vi "clear_buffers.vi"(8 "error in (no error)":errorcluster, 11 "FPGAWrapperAN110607Galvo in":refnum<class "FPGAWrapperAN110607Galvo.lvclass">) -> (0 "error out":errorcluster, 3 "FPGAWrapperAN110607Galvo out":refnum<class "FPGAWrapperAN110607Galvo.lvclass">)   [LabVIEW 2010, in "FPGAWrapperAN110607Galvo.lvclass"]
uses:
  FPGAWrapperAN110607Galvo.lvclass
  <vilib>/rvi/interface/nirviMethod/nirviMethod.xnode
  FPGA_VI_ref.ctl
  <vilib>/rvi/interface/common/niFpgaNodeNameForErrorReporting.ctl
  <vilib>/rvi/errors/niLvFpgaWhatHappensToTopLevelVI.ctl
  <vilib>/Utility/error.llb/Error Cluster From Error Code.vi
  <vilib>/rvi/errors/niLvFpgaAdjustHostInterfaceError.vi
  NiFpgaLv.dll
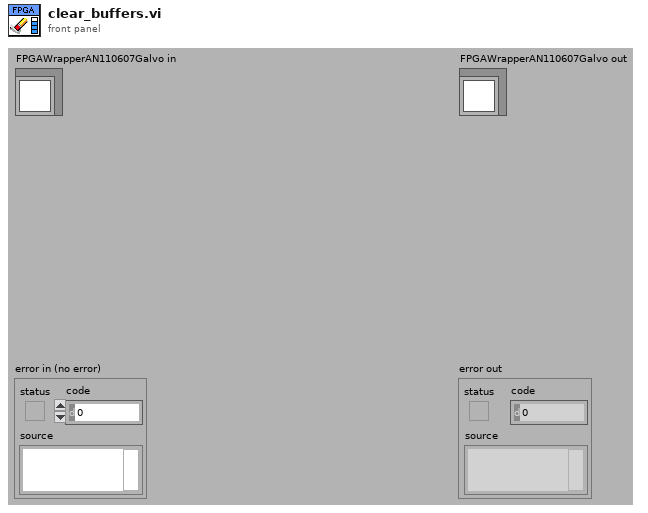
[diagram p1: front panel]
types:
  T1 = typedef "niFpgaNodeNameForErrorReporting.ctl" = enum16{"Open FPGA VI Reference", "Read/Write Control", "Invoke Method: Abort", "Invoke Method: Acknowledge IRQ", "Invoke Method: Download", "Invoke Method: FIFO.Configure", "Invoke Method: FIFO.Read", "Invoke Method: FIFO.Start", "Invoke Method: FIFO.Stop", "Invoke Method: FIFO.Write", "Invoke Method: Reset", "Invoke Method: Run", "Invoke Method: Wait on IRQ", "Close FPGA VI Reference"}
  T2 = typedef "niLvFpgaWhatHappensToTopLevelVI.ctl" = enum16{"top level VI scripted behind XNode", "top level VI inlined behind XNode"}
  T3 = typedef "FPGAWrapperAN110607Galvo.lvclass/FPGA_VI_ref.ctl" = refnum<k20>
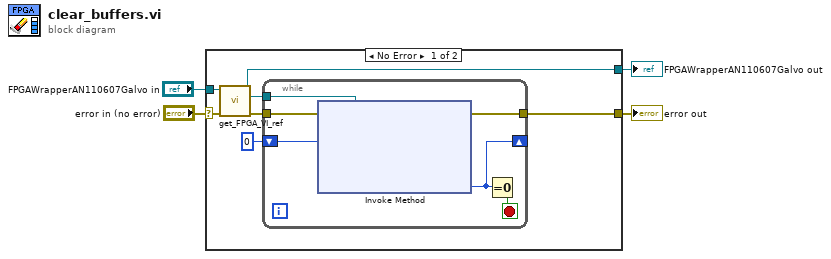
[diagram p0: block diagram]
diagram:
  n1 = case shown="No Error" "error in (no error)" {
    selector: "error in (no error)" -> [w11 w92]
    tunnel: [w6 w92] -> w3
    tunnel: "FPGAWrapperAN110607Galvo in" -> [w8 w91]
    tunnel: [w7 w91] -> w1
    frame No Error {
      n2 = call-dynamic "get_FPGA_VI_ref.vi"("error in (no error)"=w11, "FPGAWrapperAN110607Galvo in"=w8) -> ("error out"=w9:errorcluster, "FPGA VI reference"=w10:T3, "FPGAWrapperAN110607Galvo out"=w7:refnum<class "FPGAWrapperAN110607Galvo.lvclass">)  [unwired: 6 in, 1 out]
      n3 = while {
        tunnel: w10 -> [w17]
        tunnel: w9 -> [w16]
        tunnel: [w15] -> w6
        shift-right: [w12] -> _
        shift-left: u32 0 ("Elements Remaining") -> [w14]
        stop <- w13 stop-if-true
        n4 = xnode "Invoke Method"("FPGA VI Reference In"=w17, "error in"=w16, "Number of Elements"=w14) -> ("error out"=w15:errorcluster, "Elements Remaining"=w12:u32)  [unwired: 1 in, 2 out]
        n5 = Equal To 0?(x=w12) -> (x = 0?=w13:bool)
      }
    }
    frame Error {
    }
  }
  "error out" <- w3
  "FPGAWrapperAN110607Galvo out" <- w1
